vi "link -- read rusout file - cylinder.vi"(8 "rus out file path":path=path "C:/data/RUS/Experiment/ProbeTest/Probe10/YBCO_5/sweep2/9w/rusout.dat", 9 "buttons":bool[](array[boolean])=[TRUE, TRUE, TRUE, TRUE, TRUE, TRUE, TRUE, TRUE, TRUE, TRUE, TRUE, TRUE, TRUE, TRUE, TRUE, TRUE, TRUE, TRUE, TRUE, TRUE, TRUE, TRUE, TRUE, TRUE, TRUE, TRUE, TRUE, TRUE, TRUE]) -> (0 "Cluster out":T1={"freqs Exp"=[], "symmetry"=[], "dc11"=[], "freqs Fit"=[], "header"=" LANL RPRcode Ver. 6.1\r YBCO_5 93K  c11  c22  c33  c23  c13  c12\rfree moduli are  c11, c22, c33, c23, c13, c12, c44, c55,  c66\rusing 14 order polynomials   mass=     0.0016 gm  rho= 6.394 gm/cc\r \r n     fex      fr      %err  wt   k   i    df/d(moduli)\r  1 0.571390 0.570760  -0.11 1.00  4   1 -0.02 -0.07 -0.10  0.15  0.07 -0.02  0.13  0.10  0.76\r  2 0.667390 0.670743   0.50 1.00  6   2 -1.38 -9.92 -4.33 13.42 -4.20  7.28  0.13  0.01  0.00\r  3 1.010850 0.953849  -5.64 1.00  6   3 -5.51 -0.53 -6.38  1.33 12.10 -0.22  0.02  0.21  0.00\r  4 1.162310 1.153734  -0.74 1.00  2   2 -0.21 -2.72 -1.50  4.17 -0.94  1.42  0.17  0.20  0.41\r  5 1.249130 1.257304   0.65 1.00  8   2 -2.86 -0.88 -0.97 -1.10  3.20  2.97  0.18  0.19  0.28\r  6 1.628810 1.599504  -1.80 1.00  8   3 -0.18 -6.69 -5.81 12.88 -0.39  0.81  0.38  0.02  0.01\r  7 1.808600 1.811066   0.14 1.00  1   2 -0.70-10.22 -5.83 16.10 -3.98  5.51  0.00  0.00  0.13\r  8 1.877910 1.875669  -0.12 1.00  4   2 -0.61 -4.42 -1.89  5.87 -1.72  3.14  0.31  0.18  0.16\r  9 1.937090 1.921125  -0.82 1.00  6   4 -0.66 -0.50 -0.97  0.88  1.24  0.12  0.26  0.27  0.37\r 10 1.962290 1.984671   1.14 1.00  2   3 -4.07 -0.23 -2.98 -0.80  7.25  1.32  0.01  0.50  0.00\r 11 2.100020 2.053573  -2.21 1.00  5   1 -3.32-10.33 -1.97  9.33 -5.23 12.50  0.00  0.00  0.00\r 12 2.173620 2.217161   2.00 1.00  4   3 -2.73 -0.33 -2.56  0.28  5.26  0.43  0.14  0.43  0.09\r 13 2.285820 2.284220  -0.07 1.00  3   2 -0.13 -0.80 -0.88  1.62  0.20  0.08  0.00  0.00  0.90\r 14 2.339660 2.347618   0.34 1.00  7   2 -7.21 -1.26 -3.31 -3.28 10.06  5.88  0.00  0.00  0.13\r 15 2.418410 2.436259   0.74 1.00  5   2 -5.16 -5.60 -4.88  5.24  4.78  6.62  0.00  0.00  0.01\r 16 2.540360 2.578822   1.51 1.00  6   5 -0.20 -5.41 -3.77  9.33 -1.04  1.53  0.55  0.01  0.00\r 17 2.657210 2.613897  -1.63 1.00  8   4 -0.22 -1.46 -1.26  2.57  0.20  0.28  0.32  0.31  0.26\r 18 2.722880 2.698450  -0.90 1.00  2   4 -1.11 -1.96 -1.25  2.19  0.57  1.79  0.34  0.27  0.16\r 19 2.917360 2.834347  -2.85 1.00  2   5 -0.49 -2.61 -2.73  5.08  0.91  0.10  0.42  0.23  0.10\r \rBulk Modulus=    1.6521\r \r   c11     c22     c33     c23     c13     c12     c44     c55        c66\r 2.55484 2.45282 3.09885 1.25154 1.13354 1.09231 0.35620 0.30595 1.08463\r \r   d1       d2       d3\r  0.10300  0.12000  0.02050\r \r loop# 4  rms error=  1.8021 %, changed by 0.0000000 %\r \r length of gradient vector=  0.022439  blamb=  0.000000\r \r eigenvalues          eigenvectors\r      0.00000   0.11-0.29 0.47 0.18-0.69 0.05 0.37 0.10-0.09\r      0.00001   0.14-0.47-0.37 0.34 0.33 0.05 0.56-0.27-0.12\r      0.00001   0.85 0.48-0.06 0.17-0.03 0.01 0.05-0.01-0.02\r      0.05131   0.35-0.48-0.47-0.50-0.30-0.03-0.22 0.17 0.07\r      0.19574   0.31-0.31 0.64-0.39 0.48-0.03-0.01-0.12 0.03\r      0.65984   0.13-0.37 0.09 0.64 0.07-0.02-0.64 0.12 0.07\r      0.85825   0.00 0.00 0.00-0.08-0.19 0.10-0.30-0.67-0.63\r      1.86264   0.00 0.00 0.00-0.02 0.20 0.12 0.03 0.64-0.73\r      6.65340   0.00 0.00 0.00 0.03-0.02-0.98 0.04 0.00-0.17\r \rchisquare increased 2% by the following % changes in independent parameters\r************************************-10.33 -6.42  1.32\r 12.10 15.11 -2.56  6.02  4.34 12.58  5.37  2.03 -1.05\r", "bulk modulus"=0.0, "c11"=-14.16, "c22"=8.71, "free moduli"=[""], "# of polynomials"=0, "mass, g"=0.0, "density, g/cm3"=0.0, "dc22"=[], "dc33"=[], "dc23"=[], "dc13"=[], "dc12"=[], "dc44"=[], "dc55"=[], "dc66"=[], "all moduli"=[""], "c33"=0.22, "c23"=4.22, "c13"=-6.35, "c12"=-2.28, "c44"=5.66, "c55"=-5.68, "c66"=0.11, "d1"=-14.16, "d2"=8.71, "d3"=0.22, "dL11"=[], "dL12"=[], "dL22"=[], "dL33"=[], "dL44"=[], "dL55"=[], "L11"=0.0, "L12"=0.0, "L22"=0.0, "L33"=0.0, "L44"=0.0, "L55"=0.0, "# of free elastic constants"=0, "det12"=[]}, 1 "peaks exp":i32[](array[numeric])=[556, 646, 974, 1127, 1207, 1578, 1759, 1872, 1895, 2004, 2216, 2256, 2345], 2 "all peaks exp":i32[](array[numeric])=[556, 646, 974, 1127, 1207, 1578, 1759, 1872, 1895, 2004, 2216, 2256, 2345], 3 "array of coefficients":dbl[][](array[numeric]), 4 "Array of dL":dbl[][](array[numeric]), 5 "number of free elastic constants":i32=1)   [LabVIEW 2012]
uses:
  <vilib>/regexp/Match Regular Expression.xnode
  link -- rusout - tetragonal.ctl
  <vilib>/Analysis/Matrix/NI_Matrix.lvlib
  <vilib>/Analysis/Matrix/Numeric/Conversions/Array To Matrix - RA2.vi
  <vilib>/Analysis/NI_AALBase.lvlib
  <vilib>/Analysis/baseanly.llb/Real Inverse Matrix.vi
  <vilib>/Analysis/baseanly.llb/Matrix Type of Inverse Matrix.ctl
  <vilib>/Analysis/baseanly.llb/Real A x B.vi
  <vilib>/Analysis/Matrix/Numeric/Conversions/Matrix To Array - RM.vi
  <vilib>/Utility/file.llb/Read From Spreadsheet File (string).vi
panel:
  out "error":i32
  out "number of columns":i32
  out "number of rows":i32
  out "det12":dbl[](array[numeric])
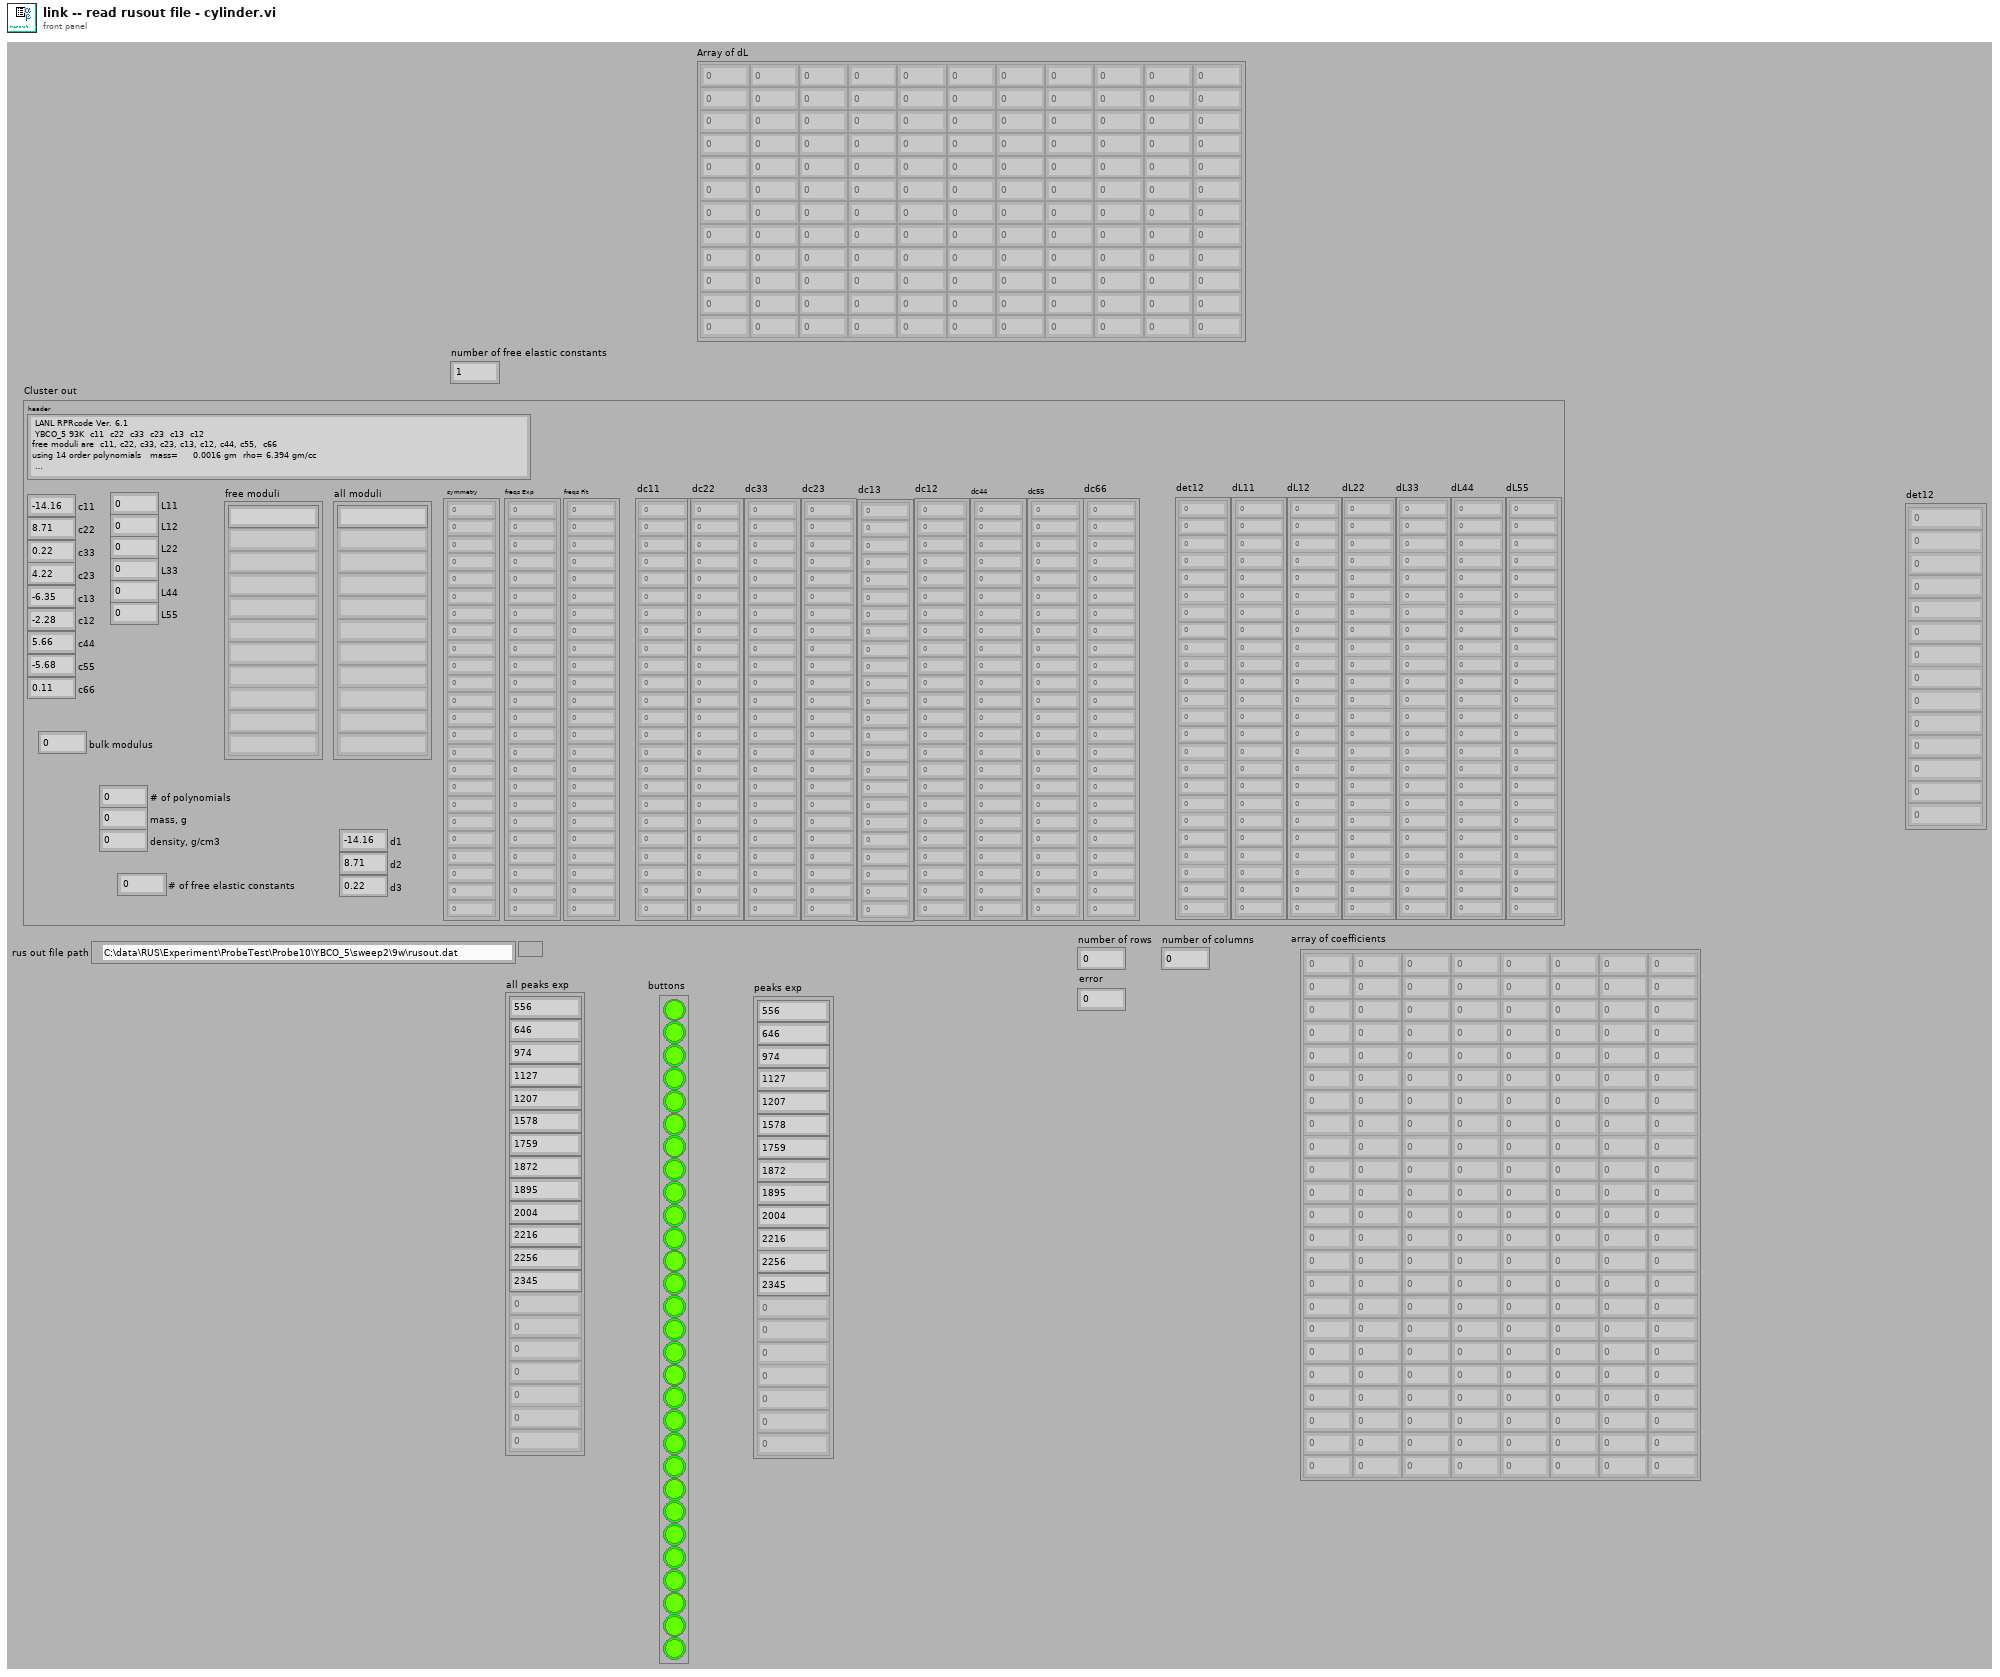
[diagram p1: front panel]
types:
  T1 = typedef "link -- rusout - tetragonal.ctl" = cluster{"freqs Exp":dbl[], "symmetry":i32[], "dc11":dbl[], "freqs Fit":dbl[], "header":string, "bulk modulus":dbl, "c11":dbl, "c22":dbl, "free moduli":string[], "# of polynomials":i32, "mass, g":dbl, "density, g/cm3":dbl, "dc22":dbl[], "dc33":dbl[], "dc23":dbl[], "dc13":dbl[], "dc12":dbl[], "dc44":dbl[], "dc55":dbl[], "dc66":dbl[], "all moduli":string[], "c33":dbl, "c23":dbl, "c13":dbl, "c12":dbl, "c44":dbl, "c55":dbl, "c66":dbl, "d1":dbl, "d2":dbl, "d3":dbl, "dL11":dbl[], "dL12":dbl[], "dL22":dbl[], "dL33":dbl[], "dL44":dbl[], "dL55":dbl[], "L11":dbl, "L12":dbl, "L22":dbl, "L33":dbl, "L44":dbl, "L55":dbl, "# of free elastic constants":i32, "det12":dbl[]}
  T2 = typedef "NI_AALBase.lvlib/Matrix Type of Inverse Matrix.ctl" = enum32{"General", "Positive Definite", "Lower Triangular", "Upper Triangular"}
  T3 = typedef "NI_Matrix.lvlib/RealMatrix.ctl" = dbl[][]
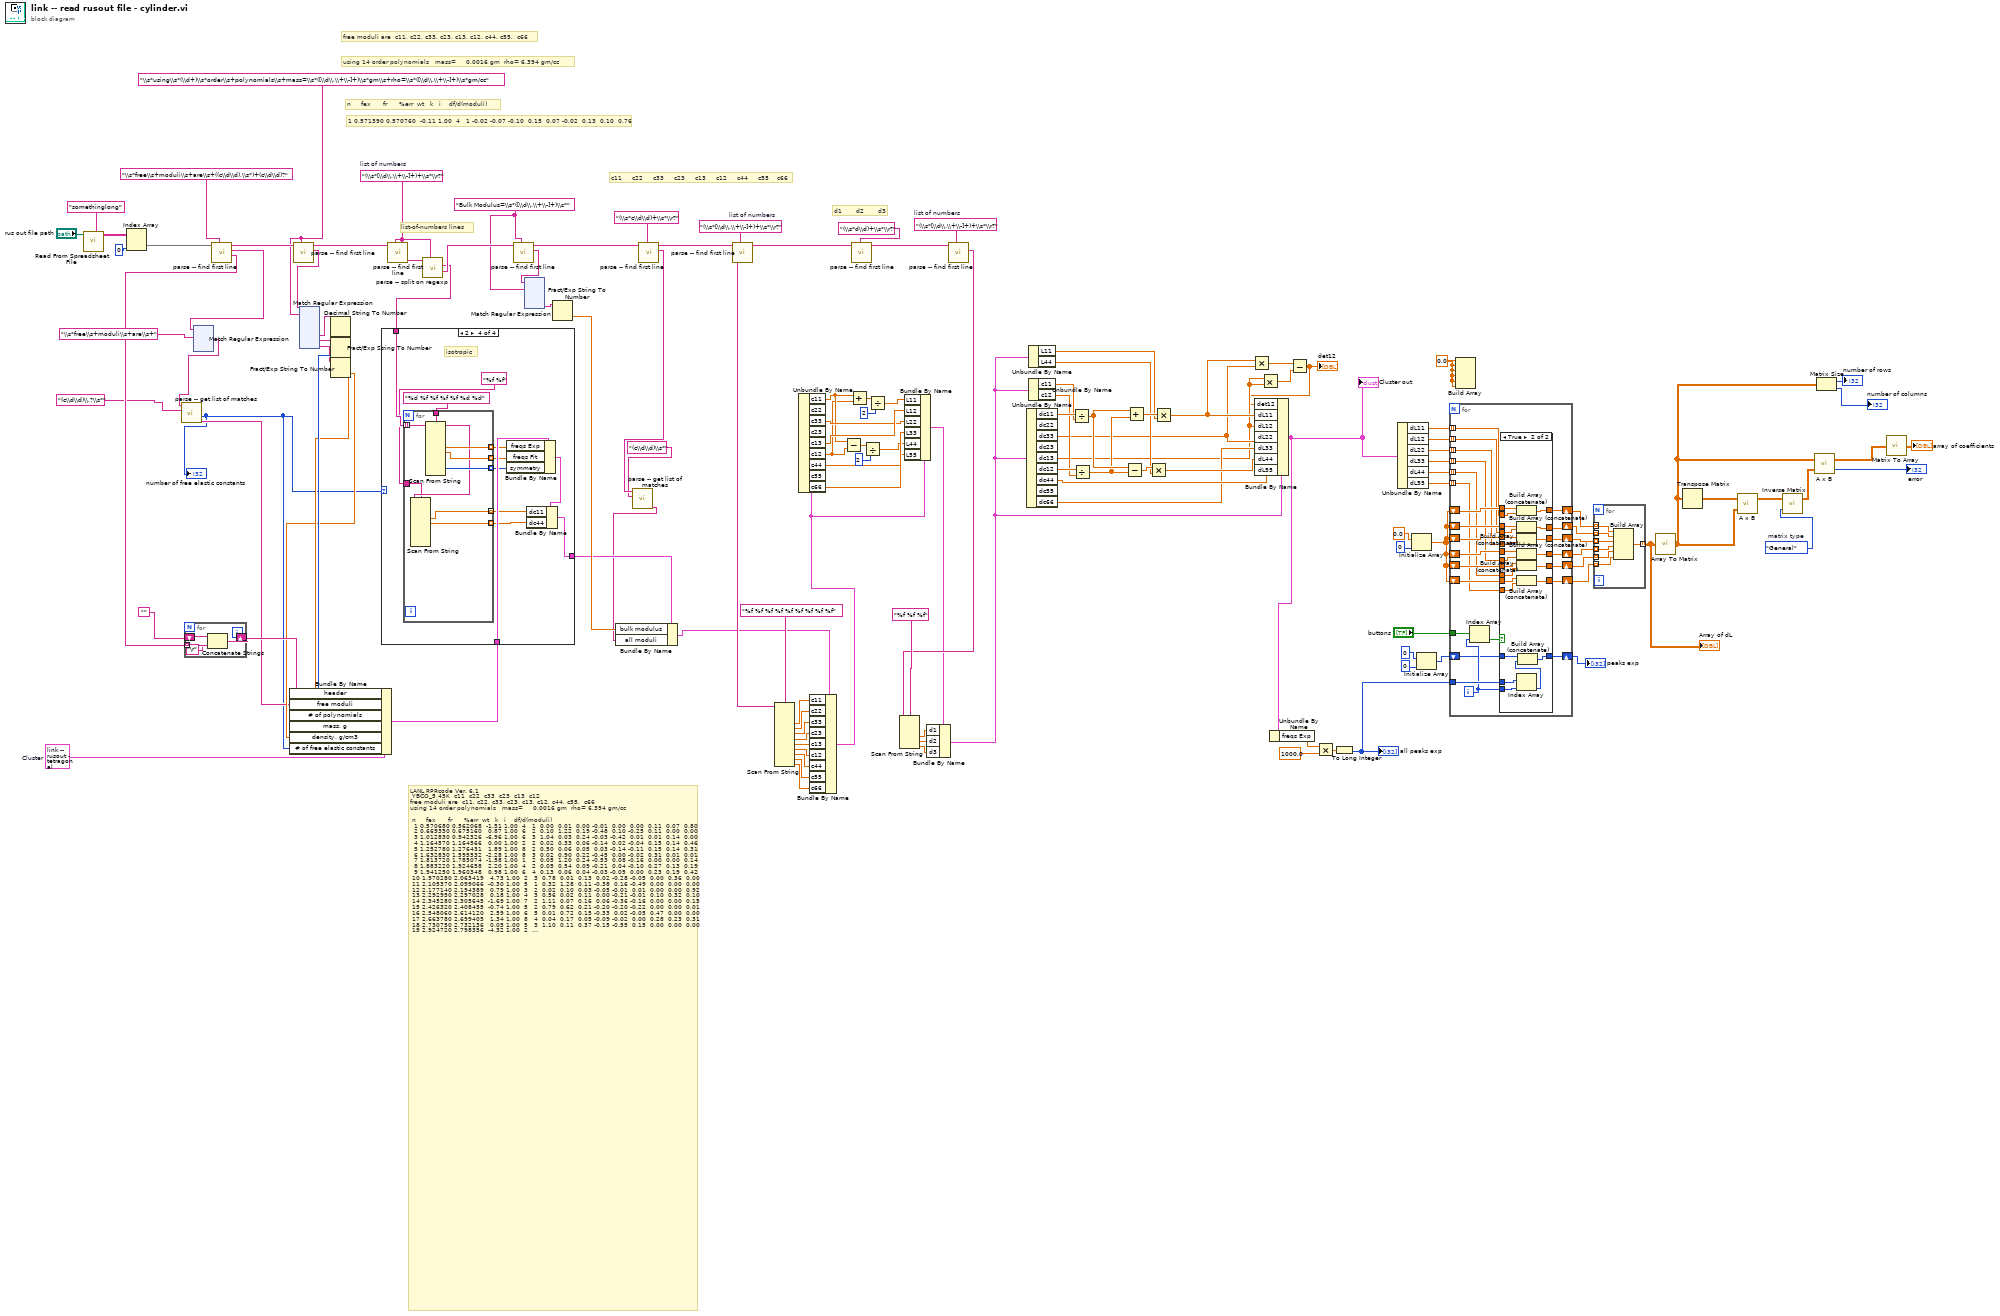
[diagram p0: block diagram]
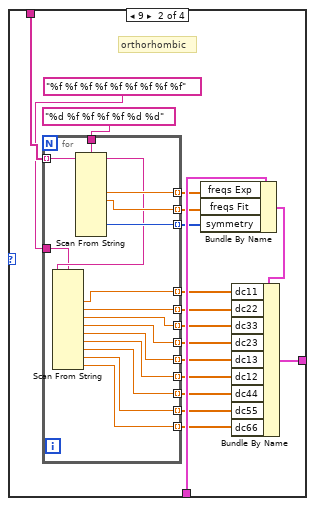
[diagram p3: hidden frame]
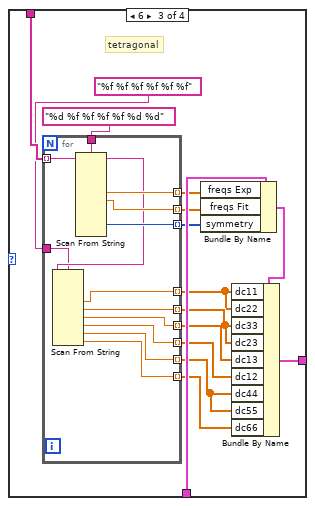
[diagram p4: hidden frame]
diagram:
  w26 = 0.0
  w43 = Matrix_Type_of_Inverse_Matrix."General"  # matrix type
  w129 = T1 {"freqs Exp"=[], "symmetry"=[], "dc11"=[], "freqs Fit"=[], "header"="", "bulk modulus"=0.0, "c11"=0.0, "c22"=0.0, "free moduli"=[], "# of polynomials"=0, "mass, g"=0.0, "density, g/cm3"=0.0, "dc22"=[], "dc33"=[], "dc23"=[], "dc13"=[], "dc12"=[], "dc44"=[], "dc55"=[], "dc66"=[], "all moduli"=[], "c33"=0.0, "c23"=0.0, "c13"=0.0, "c12"=0.0, "c44"=0.0, "c55"=0.0, "c66"=0.0, "d1"=0.0, "d2"=0.0, "d3"=0.0, "dL11"=[], "dL12"=[], "dL22"=[], "dL33"=[], "dL44"=[], "dL55"=[], "L11"=0.0, "L12"=0.0, "L22"=0.0, "L33"=0.0, "L44"=0.0, "L55"=0.0, "# of free elastic constants"=0, "det12"=[]}  # Cluster
  w113 = "\\s*using\\s*(\\d+)\\s*order\\s+polynomials\\s+mass=\\s*([\\d\\.\\+\\-]+)\\s*gm\\s+rho=\\s*([\\d\\.\\+\\-]+)\\s*gm/cc" ("format string")
  w79 = "(\\s*[\\d\\.\\+\\-]+)+\\s*\\r?"  # list of numbers
  w81 = "(\\s*[\\d\\.\\+\\-]+)+\\s*\\r?"  # list of numbers
  w101 = "Bulk Modulus=\\s*([\\d\\.\\+\\-]+)\\s*" ("format string")
  w105 = "(\\s*[\\d\\.\\+\\-]+)+\\s*\\r?"  # list of numbers
  # "LANL RPRcode Ver. 6.1\n YBCO_5 45K  c11  c22  c33  c23  c13  c12\nfree moduli are  c11, c22, c33, c23, c13, c12, c44, c55,  c66\nusing 14 order polynomials   mass=     0.0016 gm  rho= 6.394 gm/cc\n \n n     fex      fr      %err  wt   k   i    df/d(moduli)\n  1 0.570680 0.562068  -1.51 1.00  4   1  0.00  0.01  0.00 -0.01  0.00  0.00  0.11  0.07  0.80\n  2 0.669350 0.675160   0.87 1.00  6   2  0.10  1.22  0.19 -0.48  0.10 -0.25  0.11  0.00  0.00\n  3 1.012830 0.942326  -6.96 1.00  6   3  1.04  0.03  0.24 -0.03 -0.42  0.01  0.01  0.14  0.00\n  4 1.164570 1.164566   0.00 1.00  2   2  0.02  0.33  0.06 -0.14  0.02 -0.04  0.15  0.14  0.46\n  5 1.252780 1.276431   1.89 1.00  8   2  0.50  0.06  0.05  0.03 -0.14 -0.11  0.15  0.14  0.31\n  6 1.632830 1.595532  -2.28 1.00  8   3  0.02  0.90  0.22 -0.45  0.00 -0.02  0.31  0.01  0.01\n  7 1.813720 1.785074  -1.58 1.00  1   2  0.05  1.20  0.24 -0.53  0.08 -0.16  0.00  0.00  0.14\n  8 1.883220 1.924658   2.20 1.00  4   2  0.05  0.54  0.09 -0.21  0.04 -0.10  0.27  0.13  0.19\n  9 1.941250 1.960348   0.98 1.00  6   4  0.13  0.06  0.04 -0.03 -0.05  0.00  0.23  0.19  0.42\n 10 1.970280 2.063419   4.73 1.00  2   3  0.78  0.01  0.13  0.02 -0.28 -0.05  0.00  0.36  0.00\n 11 2.105370 2.099066  -0.30 1.00  5   1  0.32  1.28  0.11 -0.38  0.16 -0.49  0.00  0.00  0.00\n 12 2.177140 2.194389   0.79 1.00  3   2  0.02  0.10  0.03 -0.05 -0.01  0.01  0.00  0.00  0.92\n 13 2.292950 2.297028   0.18 1.00  4   3  0.56  0.02  0.11  0.00 -0.21 -0.01  0.10  0.32  0.10\n 14 2.345280 2.305645  -1.69 1.00  7   2  1.11  0.07  0.16  0.06 -0.36 -0.16  0.00  0.00  0.15\n 15 2.426320 2.408455  -0.74 1.00  5   2  0.79  0.62  0.21 -0.20 -0.20 -0.22  0.00  0.00  0.01\n 16 2.548060 2.614120   2.59 1.00  6   5  0.01  0.72  0.15 -0.33  0.02 -0.05  0.47  0.00  0.00\n 17 2.663780 2.699405   1.34 1.00  8   4  0.04  0.17  0.05 -0.09 -0.02  0.00  0.28  0.23  0.31\n 18 2.730750 2.732136   0.05 1.00  5   3  1.10  0.11  0.37 -0.15 -0.55  0.15  0.00  0.00  0.00\n 19 2.924720 2.798356  -4.32 1.00  2   4  0.17  0.31  0.06 -0.10 -0.01 -0.09  0.32  0.18  0.16\n \nBulk Modulus=    1.6081\n \n   c11     c22     c33     c23     c13     c12     c44     c55        c66\n 2.49397 2.44836 2.71819 1.31884 1.19770 0.96552 0.39256 0.39449 1.00088\n \n   d1       d2       d3\n  0.10300  0.12000  0.02050\n \n loop# 4  rms error=  2.5365 %, changed by 0.0000000 %\n \n length of gradient vector=  0.014672  blamb=  0.076608\n \n eigenvalues          eigenvectors\n      0.00371   0.08 0.61-0.12-0.24-0.52-0.34 0.30 0.25 0.13\n      0.02604   0.07 0.08 0.66 0.20 0.21-0.51 0.24-0.33 0.21\n      0.03278  -0.98-0.02-0.03 0.13-0.10-0.11 0.08 0.00 0.05\n      0.11472  -0.14 0.06 0.70-0.50-0.10 0.33-0.16 0.26-0.16\n      0.43786  -0.12 0.68-0.15-0.19 0.57 0.12-0.18-0.27-0.07\n      0.76749   0.05 0.39 0.22 0.75-0.23 0.37-0.15 0.11-0.09\n      0.88186   0.00 0.00 0.00-0.13-0.26 0.43 0.01-0.45 0.72\n      1.42893   0.00 0.00 0.00 0.09 0.46 0.11 0.22 0.66 0.53\n      3.81195   0.00 0.00 0.00 0.01-0.08-0.39-0.85 0.15 0.31\n \nchisquare increased 2% by the following % changes in independent parameters\n  1.11  1.00-12.66 -3.93 -3.87  2.01  0.21 -0.32  0.03\n  3.28  0.43 -0.10  0.58  8.07  5.56 -0.08 -0.10  0.02\n -0.59  3.27 -0.15  6.47 -1.59  2.77  0.01 -0.05  0.01"
  # "n     fex      fr      %err  wt   k   i    df/d(moduli)"
  # "using 14 order polynomials   mass=     0.0016 gm  rho= 6.394 gm/cc"
  # "free moduli are  c11, c22, c33, c23, c13, c12, c44, c55,  c66"
  # "d1       d2       d3"
  # "c11     c22     c33     c23     c13     c12     c44     c55    c66"
  # "list-of-numbers lines"
  # "1 0.571390 0.570760  -0.11 1.00  4   1 -0.02 -0.07 -0.10  0.15  0.07 -0.02  0.13  0.10  0.76"
  n1 = call-poly <vilib>:"Read From Spreadsheet File.vi"("delimiter (\\t)"="somethinglong" ("delimiter (\\t)"), "file path (dialog if empty)"="rus out file path") -> ("all rows"=w133:string[][])  [unwired: 5 in, 4 out]
  n2 = Index Array(array=w133, index (col)=0 ("index (row)")) -> (element=w125:string[])  [unwired: 1 in]
  n3 = call "parse -- find first line.vi"("regexp"="\\s*free\\s+moduli\\s+are\\s+((c\\d\\d),\\s*)+(c\\d\\d)?" ("format string"), "string array"=w125) -> ("before"=w124:string[], "matching line"=w115:string, "after"=w123:string[])  [unwired: 5 in, 2 out]
  n4 = for {
    tunnel: w124 -> [w139] mode=indexing
    shift-right: [w136] -> w128
    shift-left: "" -> [w137]
    n5 = Concatenate Strings(w137, w139, "\r") -> (w136:string)
  }
  n6 = xnode "Match Regular Expression"("input string"=w115, "regular expression"="\\s*free\\s+moduli\\s+are\\s+" ("format string")) -> ("after match"=w7:string)  [unwired: 4 in, 4 out]
  n7 = call "parse -- get list of matches.vi"("regexp"="(c\\d\\d)\\,?\\s*" ("format string"), "string"=w7) -> ("Array"=w6:string[], "number of free elastic constants"=w5:i32)  [unwired: 7 in, 1 out]
  "number of free elastic constants" <- w5
  n8 = call "parse -- find first line.vi"("regexp"=w113, "string array"=w123) -> ("matching line"=w114:string, "after"=w122:string[])  [unwired: 5 in, 3 out]
  n9 = xnode "Match Regular Expression"("input string"=w114, "regular expression"=w113) -> ("submatch 1"=w112:string, "submatch 2"=w110:string, "submatch 3"=w108:string)  [unwired: 4 in, 5 out]
  n10 = Decimal String To Number(string=w112) -> (number=w111:i32)  [unwired: 2 in, 1 out]
  n11 = Fract/Exp String To Number(string=w110) -> (number=w109:dbl)  [unwired: 3 in, 1 out]
  n12 = Fract/Exp String To Number(string=w108) -> (number=w107:dbl)  [unwired: 3 in, 1 out]
  n13 = Bundle By Name(cluster=w129, "header"=w128, "free moduli"=w6, "# of polynomials"=w111, "mass, g"=w109, "density, g/cm3"=w107, "# of free elastic constants"=w5) -> (w127:T1)
  n14 = call "parse -- find first line.vi"("regexp"=w105, "string array"=w122) -> ("line and after"=w106:string[])  [unwired: 5 in, 4 out]
  n15 = call "parse -- split on regexp.vi"("regexp"=w105, "string array"=w106) -> ("after"=w104:string[], "matching lines"=w103:string[])  [unwired: 7 in, 1 out]
  n16 = case shown="2" w5 {
    tunnel: w127 -> [w140 w157 w188 w212]
    tunnel: w103 -> [_ w156 w187 w211]
    tunnel: [w140 w141 w181 w205] -> w98
    frame 0, Default {
    }
    frame 9 {
      # "orthorhombic"
      n17 = for {
        tunnel: "%d %f %f %f %f %d %d" ("format string") -> [w174]
        tunnel: w156 -> [w173] mode=indexing
        tunnel: [w172] -> w155 mode=indexing
        tunnel: [w171] -> w154 mode=indexing
        tunnel: [w170] -> w153 mode=indexing
        tunnel: "%f %f %f %f %f %f %f %f %f" ("format string") -> [w168]
        tunnel: [w167] -> w150 mode=indexing
        tunnel: [w166] -> w149 mode=indexing
        tunnel: [w165] -> w148 mode=indexing
        tunnel: [w164] -> w147 mode=indexing
        tunnel: [w163] -> w146 mode=indexing
        tunnel: [w162] -> w145 mode=indexing
        tunnel: [w161] -> w144 mode=indexing
        tunnel: [w160] -> w143 mode=indexing
        tunnel: [w159] -> w142 mode=indexing
        n18 = Scan From String(format string=w174, input string=w173) -> (remaining string=w169:string, output 2=w172:dbl, output 3=w171:dbl, output 6=w170:i32)  [unwired: 13 in, 2 out]
        n19 = Scan From String(format string=w168, input string=w169) -> (output 1=w167:dbl, output 2=w166:dbl, output 3=w165:dbl, output 4=w164:dbl, output 5=w163:dbl, output 6=w162:dbl, output 7=w161:dbl, output 8=w160:dbl, output 9=w159:dbl)  [unwired: 11 in, 3 out]
      }
      n20 = Bundle By Name(cluster=w157, "freqs Exp"=w155, "freqs Fit"=w154, "symmetry"=w153) -> (w151:T1)
      n21 = Bundle By Name(cluster=w151, "dc11"=w150, "dc22"=w149, "dc33"=w148, "dc23"=w147, "dc13"=w146, "dc12"=w145, "dc44"=w144, "dc55"=w143, "dc66"=w142) -> (w141:T1)
    }
    frame 6 {
      # "tetragonal"
      n22 = for {
        tunnel: "%d %f %f %f %f %d %d" ("format string") -> [w202]
        tunnel: w187 -> [w201] mode=indexing
        tunnel: [w200] -> w186 mode=indexing
        tunnel: [w199] -> w185 mode=indexing
        tunnel: [w198] -> w184 mode=indexing
        tunnel: "%f %f %f %f %f %f" ("format string") -> [w196]
        tunnel: [w195] -> w175 mode=indexing
        tunnel: [w194] -> w176 mode=indexing
        tunnel: [w193] -> w180 mode=indexing
        tunnel: [w192] -> w179 mode=indexing
        tunnel: [w191] -> w177 mode=indexing
        tunnel: [w190] -> w178 mode=indexing
        n23 = Scan From String(format string=w202, input string=w201) -> (remaining string=w197:string, output 2=w200:dbl, output 3=w199:dbl, output 6=w198:i32)  [unwired: 13 in, 2 out]
        n24 = Scan From String(format string=w196, input string=w197) -> (output 1=w195:dbl, output 2=w194:dbl, output 3=w193:dbl, output 4=w192:dbl, output 5=w191:dbl, output 6=w190:dbl)  [unwired: 8 in, 3 out]
      }
      n25 = Bundle By Name(cluster=w188, "freqs Exp"=w186, "freqs Fit"=w185, "symmetry"=w184) -> (w182:T1)
      n26 = Bundle By Name(cluster=w182, "dc11"=w175, "dc22"=w175, "dc33"=w176, "dc23"=w176, "dc13"=w180, "dc12"=w179, "dc44"=w177, "dc55"=w177, "dc66"=w178) -> (w181:T1)
    }
    frame 2 {
      # "isotropic"
      n27 = for {
        tunnel: "%d %f %f %f %f %d %d" ("format string") -> [w222]
        tunnel: w211 -> [w221] mode=indexing
        tunnel: [w220] -> w210 mode=indexing
        tunnel: [w219] -> w209 mode=indexing
        tunnel: [w218] -> w208 mode=indexing
        tunnel: "%f %f" ("format string") -> [w216]
        tunnel: [w215] -> w203 mode=indexing
        tunnel: [w214] -> w204 mode=indexing
        n28 = Scan From String(format string=w222, input string=w221) -> (remaining string=w217:string, output 2=w220:dbl, output 3=w219:dbl, output 6=w218:i32)  [unwired: 13 in, 2 out]
        n29 = Scan From String(format string=w216, input string=w217) -> (output 1=w215:dbl, output 2=w214:dbl)  [unwired: 12 in, 3 out]
      }
      n30 = Bundle By Name(cluster=w212, "freqs Exp"=w210, "freqs Fit"=w209, "symmetry"=w208) -> (w206:T1)
      n31 = Bundle By Name(cluster=w206, "dc11"=w203, "dc44"=w204) -> (w205:T1)
    }
  }
  n32 = call "parse -- find first line.vi"("regexp"=w101, "string array"=w104) -> ("matching line"=w102:string, "after"=w121:string[])  [unwired: 5 in, 3 out]
  n33 = xnode "Match Regular Expression"("input string"=w102, "regular expression"=w101) -> ("submatch 1"=w100:string)  [unwired: 4 in, 5 out]
  n34 = Fract/Exp String To Number(string=w100) -> (number=w99:dbl)  [unwired: 3 in, 1 out]
  n35 = call "parse -- find first line.vi"("regexp"="(\\s*c\\d\\d)+\\s*\\r?" ("format string"), "string array"=w121) -> ("matching line"=w4:string, "after"=w120:string[])  [unwired: 5 in, 3 out]
  n36 = call "parse -- get list of matches.vi"("regexp"="(c\\d\\d)\\s*" ("format string"), "string"=w4) -> ("Array"=w2:string[])  [unwired: 7 in, 2 out]
  n37 = Bundle By Name(cluster=w98, "bulk modulus"=w99, "all moduli"=w2) -> (w87:T1)
  n38 = call "parse -- find first line.vi"("regexp"=w81, "string array"=w120) -> ("matching line"=w97:string, "after"=w119:string[])  [unwired: 5 in, 3 out]
  n39 = Scan From String(format string="%f %f %f %f %f %f %f %f %f", input string=w97) -> (output 1=w96:dbl, output 2=w95:dbl, output 3=w94:dbl, output 4=w93:dbl, output 5=w92:dbl, output 6=w91:dbl, output 7=w90:dbl, output 8=w89:dbl, output 9=w88:dbl)  [unwired: 11 in, 3 out]
  n40 = Bundle By Name(cluster=w87, "c11"=w96, "c22"=w95, "c33"=w94, "c23"=w93, "c13"=w92, "c12"=w91, "c44"=w90, "c55"=w89, "c66"=w88) -> (w66:T1)
  n41 = Unbundle By Name(w66) -> ("c11"=w70:dbl, "c33"=w74:dbl, "c13"=w75:dbl, "c12"=w69:dbl, "c44"=w72:dbl, "c66"=w73:dbl)  [unwired: 3 out]
  n42 = Subtract(x=w70, y=w69) -> (x-y=w71:dbl)
  n43 = Add(x=w70, y=w69) -> (x+y=w78:dbl)
  n44 = call "parse -- find first line.vi"("regexp"="(\\s*d\\d)+\\s*\\r?" ("format string"), "string array"=w119) -> ("after"=w118:string[])  [unwired: 5 in, 4 out]
  n45 = Divide(x=w71, y=2) -> (x/y=w67:dbl)
  n46 = Divide(x=w78, y=2) -> (x/y=w76:dbl)
  n47 = Bundle By Name(cluster=w66, "L11"=w76, "L12"=w75, "L22"=w74, "L33"=w73, "L44"=w67, "L55"=w72) -> (w65:T1)
  n48 = call "parse -- find first line.vi"("regexp"=w79, "string array"=w118) -> ("matching line"=w83:string)  [unwired: 5 in, 4 out]
  n49 = Scan From String(format string="%f %f %f", input string=w83) -> (output 1=w86:dbl, output 2=w85:dbl, output 3=w84:dbl)  [unwired: 5 in, 3 out]
  n50 = Bundle By Name(cluster=w65, "d1"=w86, "d2"=w85, "d3"=w84) -> (w60:T1)
  n51 = Unbundle By Name(w60) -> ("dc11"=w64:dbl[], "dc33"=w49:dbl[], "dc13"=w48:dbl[], "dc12"=w62:dbl[], "dc44"=w52:dbl[], "dc66"=w51:dbl[])  [unwired: 3 out]
  n52 = Unbundle By Name(w60) -> ("L11"=w58:dbl, "L44"=w54:dbl)
  n53 = Unbundle By Name(w60) -> ("c11"=w63:dbl, "c12"=w61:dbl)
  n54 = Divide(x=w64, y=w63) -> (x/y=w57:dbl[])
  n55 = Divide(x=w62, y=w61) -> (x/y=w56:dbl[])
  n56 = Subtract(x=w57, y=w56) -> (x-y=w55:dbl[])
  n57 = Add(x=w57, y=w56) -> (x+y=w59:dbl[])
  n58 = Multiply(x=w55, y=w54) -> (x*y=w53:dbl[])
  n59 = Multiply(x=w59, y=w58) -> (x*y=w50:dbl[])
  n60 = Multiply(x=w50, y=w49) -> (x*y=w47:dbl[])
  n61 = Multiply(x=w48, y=w48) -> (x*y=w46:dbl[])
  n62 = Subtract(x=w47, y=w46) -> (x-y=w1:dbl[])
  "det12" <- w1
  n63 = Bundle By Name(cluster=w60, "det12"=w1, "dL11"=w50, "dL12"=w48, "dL22"=w49, "dL33"=w51, "dL44"=w53, "dL55"=w52) -> (w14:T1)
  "Cluster out" <- w14
  n64 = Unbundle By Name(w14) -> ("freqs Exp"=w16:dbl[])
  n65 = Multiply(x=w16, y=1000.0) -> (x*y=w15:dbl[])
  n66 = To Long Integer(number=w15) -> (32bit integer=w11:i32[])
  "all peaks exp" <- w11
  n67 = Unbundle By Name(w14) -> ("dL11"=w42:dbl[], "dL12"=w41:dbl[], "dL22"=w40:dbl[], "dL33"=w39:dbl[], "dL44"=w38:dbl[], "dL55"=w37:dbl[])
  n68 = Initialize Array(0.0, 0) -> (w25:dbl[])
  n69 = Initialize Array(0, 0) -> (w10:i32[])
  n70 = for {
    tunnel: w42 -> [w233] mode=indexing
    tunnel: w41 -> [w232] mode=indexing
    tunnel: w40 -> [w231] mode=indexing
    tunnel: w39 -> [w230] mode=indexing
    tunnel: w38 -> [w229] mode=indexing
    tunnel: w37 -> [w228] mode=indexing
    tunnel: "buttons" -> [w246]
    shift-right: [w227] -> w22
    shift-left: w25 -> [w245]
    shift-right: [w235] -> w24
    shift-left: w25 -> [w234]
    shift-right: [w236] -> w23
    shift-left: w25 -> [w237]
    shift-right: [w238] -> w21
    shift-left: w25 -> [w239]
    shift-right: [w241] -> w20
    shift-left: w25 -> [w240]
    shift-right: [w242] -> w19
    shift-left: w25 -> [w243]
    tunnel: w11 -> [w226]
    shift-right: [w223] -> w9
    shift-left: w10 -> [w224]
    i -> [w225]
    n71 = Index Array(array=w246, index=w225) -> (element=w244:bool)
    n72 = case shown="True" w244 {
      tunnel: w245 -> [w251 w276]
      tunnel: [w251 w275] -> w227
      tunnel: w243 -> [w248 w274]
      tunnel: [w248 w273] -> w242
      tunnel: [w249 w272] -> w241
      tunnel: w240 -> [w249 w271]
      tunnel: w239 -> [w250 w270]
      tunnel: [w250 w269] -> w238
      tunnel: w237 -> [w252 w268]
      tunnel: [w252 w267] -> w236
      tunnel: [w253 w266] -> w235
      tunnel: w234 -> [w253 w265]
      tunnel: w233 -> [_ w264]
      tunnel: w232 -> [_ w263]
      tunnel: w231 -> [_ w262]
      tunnel: w230 -> [_ w261]
      tunnel: w229 -> [_ w260]
      tunnel: w228 -> [_ w259]
      tunnel: w226 -> [_ w258]
      tunnel: w225 -> [_ w257]
      tunnel: w224 -> [w247 w256]
      tunnel: [w247 w255] -> w223
      frame False {
      }
      frame True {
        n73 = Build Array (concatenate)(w265, w264) -> (w266:dbl[])
        n74 = Build Array (concatenate)(w268, w263) -> (w267:dbl[])
        n75 = Build Array (concatenate)(w276, w262) -> (w275:dbl[])
        n76 = Build Array (concatenate)(w270, w261) -> (w269:dbl[])
        n77 = Build Array (concatenate)(w271, w260) -> (w272:dbl[])
        n78 = Build Array (concatenate)(w274, w259) -> (w273:dbl[])
        n79 = Index Array(array=w258, index=w257) -> (element=w254:i32)
        n80 = Build Array (concatenate)(w256, w254) -> (w255:i32[])
      }
    }
  }
  "peaks exp" <- w9
  n81 = Build Array(w26, w26, w26, w26, w26, w26) -> ()  [unwired: 1 out]
  n82 = for {
    tunnel: w24 -> [w283] mode=indexing
    tunnel: w23 -> [w282] mode=indexing
    tunnel: w22 -> [w281] mode=indexing
    tunnel: w21 -> [w280] mode=indexing
    tunnel: w20 -> [w279] mode=indexing
    tunnel: w19 -> [w278] mode=indexing
    tunnel: [w277] -> w18 mode=indexing
    n83 = Build Array(w283, w282, w281, w280, w279, w278) -> (w277:dbl[])
  }
  "Array of dL" <- w18
  n84 = call-poly <vilib>:"Array To Matrix.vi"("Real 2D Array"=w18) -> ("Real Matrix"=w30:T3)
  n85 = Transpose Matrix(1:w30) -> (0:w31:T3)
  n86 = call-poly <vilib>:"A x B.vi"("B"=w30, "A"=w31) -> ("A x B"=w29:T3)  [unwired: 1 out]
  n87 = call-poly <vilib>:"Inverse Matrix.vi"("matrix type"=w43, "Input Matrix"=w29) -> ("Inverse Matrix"=w28:T3)  [unwired: 1 out]
  n88 = call-poly <vilib>:"A x B.vi"("B"=w28, "A"=w30) -> ("error"=→"error":i32, "A x B"=w34:T3)
  n89 = Matrix Size(0:w30) -> (1:→"number of rows":i32, 2:→"number of columns":i32)
  n90 = call-poly <vilib>:"Matrix To Array.vi"("Real Matrix"=w34) -> ("Real 2D Array"=→"array of coefficients":dbl[][])
